vi "Batch_Create Waveforms.vi"() -> ()   [LabVIEW 2013]
uses:
  <vilib>/Utility/file.llb/Read From Spreadsheet File (string).vi
panel:
  in  "Waveform Definition File":path=path "C:/Users/user/Documents/AD2240/Waveforms/RFFE6"
  in  "SetID Pin State":u8(ring) items=["0", "1", "Z"]
  in  "Mode":enum16{"Write", "Read"}(ring)
  in  "Waveform file path":path=path "C:/Users/user/Documents/AD2240/Waveforms/RFFE6"
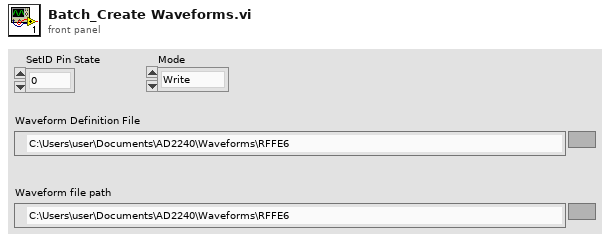
[diagram p1: front panel]
types:
  T1 = cluster{"Slave Address":u8, "Register":u8, "Data":u8}
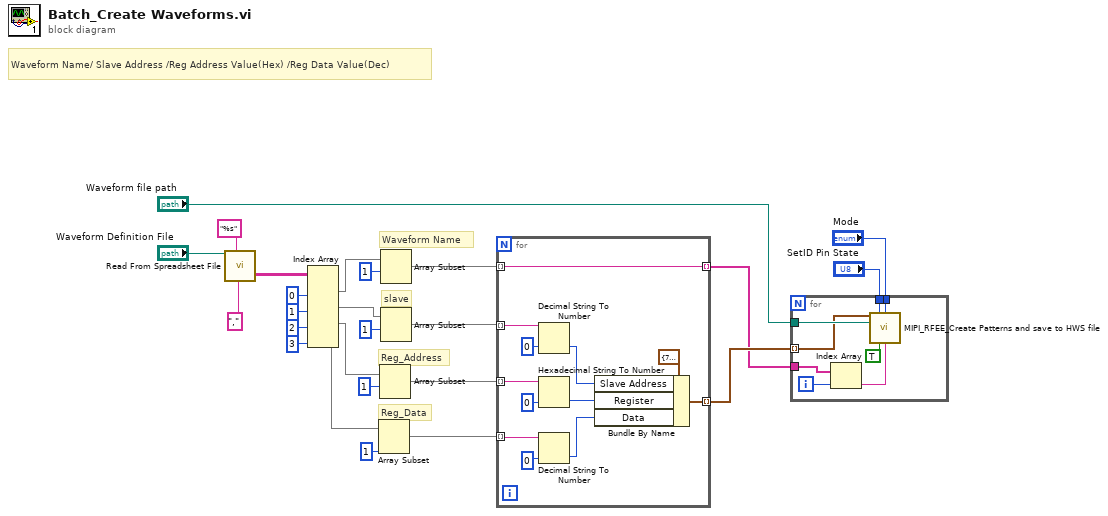
[diagram p0: block diagram]
diagram:
  # "Reg_Data"
  # "Reg_Address"
  # "slave"
  # "Waveform Name"
  # "Waveform Name/\tSlave Address\t/Reg Address Value(Hex)\t/Reg Data Value(Dec)"
  n1 = call-poly <vilib>:"Read From Spreadsheet File.vi"("delimiter (\\t)"="," ("delimiter (\\t)"), "format (%s)"="%s", "file path (dialog if empty)"="Waveform Definition File") -> ("all rows"=w21:string[][])  [unwired: 4 in, 4 out]
  n2 = Index Array(array=w21, index (col) #1=0 ("disabled index (col)"), index (col) #2=1 ("index (col)"), index (col) #3=2 ("index (col)"), index (col) #4=3 ("index (col)")) -> (element #1=w16:string[], element #2=w12:string[], element #3=w9:string[], element #4=w5:string[])  [unwired: 4 in]
  n3 = Array Subset(array=w5, index=1) -> (w4:string[])  [unwired: 1 in]
  n4 = Array Subset(array=w9, index=1) -> (w8:string[])  [unwired: 1 in]
  n5 = Array Subset(array=w16, index=1) -> (w14:string[])  [unwired: 1 in]
  n6 = Array Subset(array=w12, index=1) -> (w13:string[])  [unwired: 1 in]
  n7 = for {
    tunnel: w14 -> [w29] mode=indexing
    tunnel: w13 -> [w31] mode=indexing
    tunnel: [w32] -> w3 mode=indexing
    tunnel: w8 -> [w30] mode=indexing
    tunnel: [w29] -> w2 mode=indexing
    tunnel: w4 -> [w28] mode=indexing
    n8 = Decimal String To Number(string=w31, default (0L)=u8 0 ("Slave Address")) -> (number=w33:u8)  [unwired: 1 in, 1 out]
    n9 = Hexadecimal String To Number(string=w30, default (0uL)=u8 0 ("Register")) -> (number=w35:u8)  [unwired: 1 in, 1 out]
    n10 = Decimal String To Number(string=w28, default (0L)=u8 0 ("Data")) -> (number=w26:u8)  [unwired: 1 in, 1 out]
    n11 = Bundle By Name(cluster=T1 {"Slave Address"=7, "Register"=65, "Data"=3} ("Register Read/Write"), "Slave Address"=w33, "Register"=w35, "Data"=w26) -> (w32:T1)
  }
  n12 = for {
    tunnel: "Waveform file path" -> [w45]
    tunnel: "Mode" -> [w44]
    tunnel: "SetID Pin State" -> [w43]
    tunnel: w3 -> [w42] mode=indexing
    tunnel: w2 -> [w40]
    i -> [w41]
    n13 = Index Array(array=w40, index=w41) -> (element=w39:string)
    n14 = call "MIPI_RFEE_Create Patterns and save to HWS file.vi"("Register Read/Write"=w42, "SetID Pin State"=w43, "Mode"=w44, "file path"=w45, "Save .HWS?"=TRUE, "Filename"=w39) -> ()  [unwired: 10 in]
  }
